vi "ReadDTCs.vi"(8 "error in (no error)":errorcluster, 9 "timeout ms (1000)":u32=1000, 10 "Options (KWP/UDS Only)":T1, 11 "Ref":T4) -> (0 "error out":errorcluster, 2 "Active DTCs":T3[](array[typedef]), 3 "Ref":T4)   [LabVIEW 2015, in "Diagnostics Host Automation API.lvlib"]
uses:
  Diagnostics Host Automation API.lvlib
  Shared/Types/HostAutomation.Ref.ctl
  <vilib>/NI/STM/TCP/TCP Connection Info.ctl
  <vilib>/NI/STM/SubVIs/MetaDataElement.ctl
  Shared/Types/DTC.Codes.ctl
  Shared/Types/Command.ReadDTC.DTCs.ctl
  Shared/Types/Command.ReadDTC.ctl
  Shared/Types/DTC.Descriptor.Override.ctl
  Shared/Types/DTC.Info.ctl
  Shared/Diagnostics Addon Shared.lvlib
  <vilib>/NI/NIVS Addon Network Comm/Shared/NI VeriStand Addon Network Comm Shared.lvlib
  <vilib>/NI/STM/NI STM.lvlib
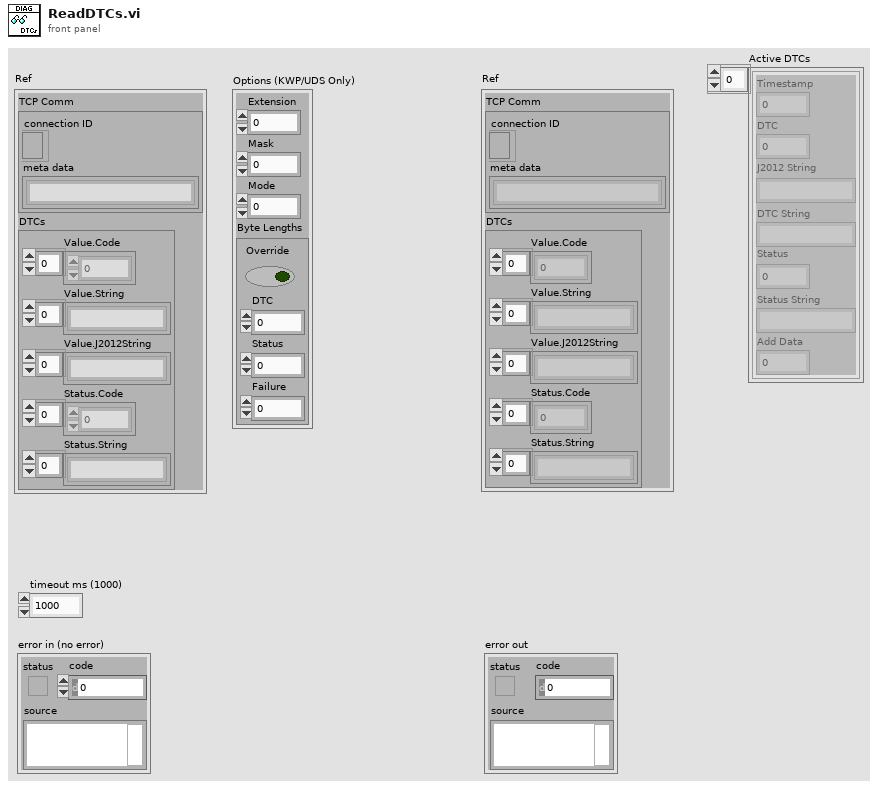
[diagram p1: front panel]
types:
  T1 = typedef "Diagnostics Addon Shared.lvlib/Command.ReadDTC.ctl" = cluster{"Extension":u32, "Mask":u32, "Mode":u32, "Byte Lengths":T2}
  T2 = typedef "Diagnostics Addon Shared.lvlib/DTC.Descriptor.Override.ctl" = cluster{"Override":bool, "DTC":u32, "Status":u32, "Failure":u32}
  T3 = typedef "Diagnostics Addon Shared.lvlib/Command.ReadDTC.DTCs.ctl" = cluster{"Timestamp":dbl, "DTC":dbl, "J2012 String":string, "DTC String":string, "Status":dbl, "Status String":string, "Add Data":dbl}
  T4 = typedef "Diagnostics Addon Shared.lvlib/HostAutomation.Ref.ctl" = cluster{"TCP Comm":T5, "DTCs":T7}
  T5 = typedef "NI STM.lvlib/TCP Connection Info.ctl" = cluster{"connection ID":refnum<k5>, "meta data":T6[]}
  T6 = typedef "NI STM.lvlib/MetaDataElement.ctl" = string
  T7 = typedef "Diagnostics Addon Shared.lvlib/DTC.Codes.ctl" = cluster{"Value.Code":dbl[], "Value.String":string[], "Value.J2012String":string[], "Status.Code":dbl[], "Status.String":string[]}
  T8 = typedef "Diagnostics Addon Shared.lvlib/DTC.Info.ctl" = cluster{"Timestamp":dbl, "DTC":dbl, "Status":dbl, "Add Data":dbl}
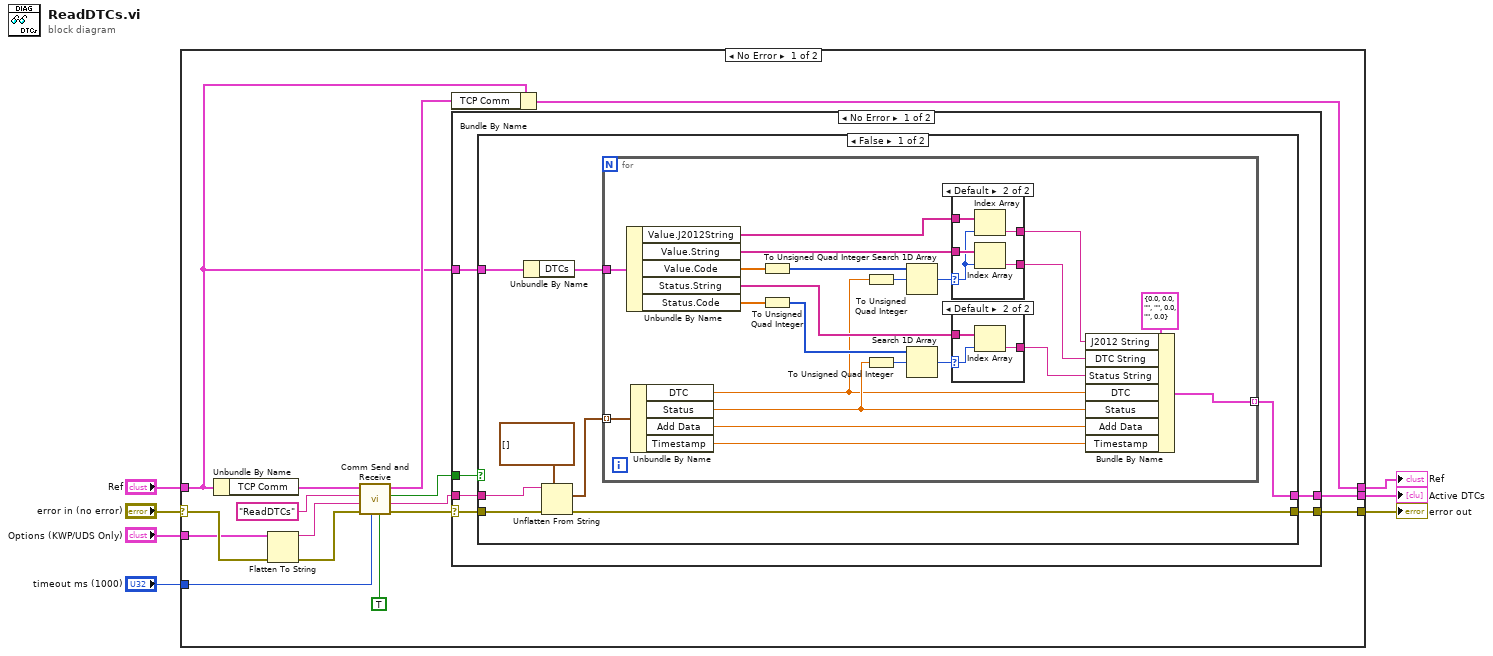
[diagram p0: block diagram]
diagram:
  n1 = case shown="No Error" "error in (no error)" {
    selector: "error in (no error)" -> [w21 w71]
    tunnel: "Ref" -> [w8 w70]
    tunnel: [w9 w70] -> w6
    tunnel: [w23 w71] -> w5
    tunnel: "timeout ms (1000)" -> [w12 _]
    tunnel: [w22 _] -> w2
    tunnel: "Options (KWP/UDS Only)" -> [w20 _]
    frame No Error {
      n2 = Unbundle By Name(w8) -> ("TCP Comm"=w11:T5)
      n3 = Flatten To String(anything=w20, error in (no error)=w21) -> (data string=w18:string, error out=w14:errorcluster)  [unwired: 2 in, 1 out]
      n4 = call <vilib>:"Comm Send and Receive.vi"("Resp Required?"=TRUE, "Timeout (ms)"=w12, "error in (no error)"=w14, "Data"=w18, "Name"="ReadDTCs", "connection info"=w11) -> ("error out"=w16:errorcluster, "Data"=w15:string, "Timed Out?"=w17:bool, "connection info"=w10:T5)  [unwired: 2 in]
      n5 = Bundle By Name(cluster=w8, "TCP Comm"=w10) -> (w9:T4)
      n6 = case shown="No Error" w16 {
        selector: w16 -> [w27 w69]
        tunnel: w17 -> [w29 _]
        tunnel: [w28 w69] -> w23
        tunnel: w15 -> [w26 _]
        tunnel: [w25 _] -> w22
        tunnel: w8 -> [w24 _]
        frame No Error {
          n7 = case shown="False" w29 {
            tunnel: [w36 w68] -> w28
            tunnel: w27 -> [w37 w68]
            tunnel: w26 -> [w34 _]
            tunnel: [w30 _] -> w25
            tunnel: w24 -> [w33 _]
            frame False {
              n8 = Unbundle By Name(w33) -> ("DTCs"=w32:T7)
              n9 = Unflatten From String(type=T8[] [] ("Active DTCs"), binary string=w34, error in (no error)=w37) -> (value=w31:T8[], error out=w36:errorcluster)  [unwired: 2 in, 1 out]
              n10 = for {
                tunnel: w31 -> [w59] mode=indexing
                tunnel: w32 -> [w58]
                tunnel: [w40] -> w30 mode=indexing
                n11 = Unbundle By Name(w58) -> ("Value.J2012String"=w39:string[], "Value.String"=w55:string[], "Value.Code"=w57:dbl[], "Status.String"=w52:string[], "Status.Code"=w53:dbl[])
                n12 = Unbundle By Name(w59) -> ("DTC"=w43:dbl, "Status"=w44:dbl, "Add Data"=w45:dbl, "Timestamp"=w46:dbl)
                n13 = To Unsigned Quad Integer(1:w57) -> (0:w51:u64[])
                n14 = To Unsigned Quad Integer(1:w53) -> (0:w50:u64[])
                n15 = To Unsigned Quad Integer(1:w43) -> (0:w48:u64)
                n16 = To Unsigned Quad Integer(1:w44) -> (0:w49:u64)
                n17 = Search 1D Array(1D array=w51, element=w48) -> (index of element=w56:i32)  [unwired: 1 in]
                n18 = Search 1D Array(1D array=w50, element=w49) -> (index of element=w54:i32)  [unwired: 1 in]
                n19 = case shown="Default" w56 {
                  selector: w56 -> [_ w64]
                  tunnel: w55 -> [_ w67]
                  tunnel: [_ w66] -> w41
                  tunnel: w39 -> [_ w65]
                  tunnel: [_ w63] -> w38
                  frame -1 {
                  }
                  frame Default {
                    n20 = Index Array(array=w65, index=w64) -> (element=w63:string)
                    n21 = Index Array(array=w67, index=w64) -> (element=w66:string)
                  }
                }
                n22 = case shown="Default" w54 {
                  selector: w54 -> [_ w61]
                  tunnel: w52 -> [_ w62]
                  tunnel: [_ w60] -> w42
                  frame -1 {
                  }
                  frame Default {
                    n23 = Index Array(array=w62, index=w61) -> (element=w60:string)
                  }
                }
                n24 = Bundle By Name(cluster=T3 {"Timestamp"=0.0, "DTC"=0.0, "J2012 String"="", "DTC String"="", "Status"=0.0, "Status String"="", "Add Data"=0.0} ("Diagnostic Trouble Code"), "J2012 String"=w38, "DTC String"=w41, "Status String"=w42, "DTC"=w43, "Status"=w44, "Add Data"=w45, "Timestamp"=w46) -> (w40:T3)
              }
            }
            frame True {
            }
          }
        }
        frame Error {
        }
      }
    }
    frame Error {
    }
  }
  "Ref" <- w6
  "error out" <- w5
  "Active DTCs" <- w2
